vi "crop_with_offset.vi"(0 "Out Rows":i32, 2 "Array":i32[][](array[numeric]), 5 "Out Cols":i32, 9 "Offset X":i32, 11 "Offset Y":i32) -> (4 "subarray":i32[][](array[numeric]))   [LabVIEW 2024]
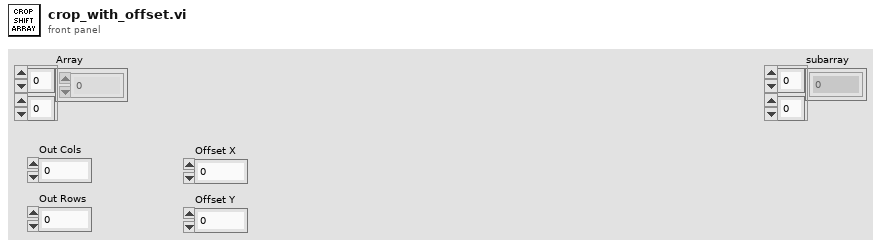
[diagram p1: front panel]
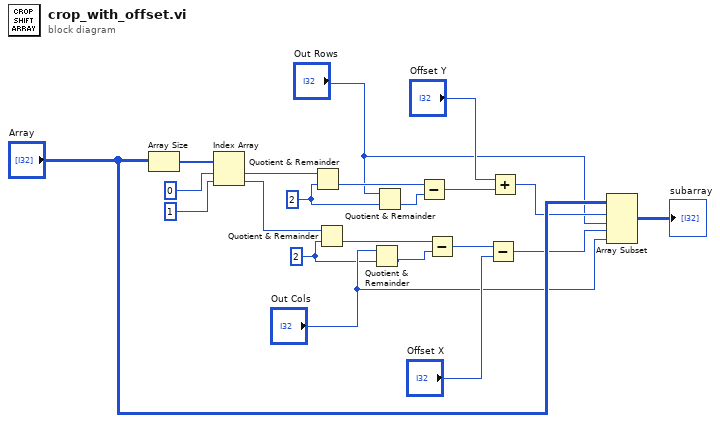
[diagram p0: block diagram]
diagram:
  w2 = 2
  w5 = 2
  n1 = Array Size(array="Array") -> (size(s)=w21:i32[])
  n2 = Index Array(array=w21, index #1=0 ("index"), index #2=1 ("index")) -> (element #1=w18:i32, element #2=w17:i32)
  n3 = Quotient & Remainder(x=w18, y=w5) -> (floor(x/y)=w16:i32)  [unwired: 1 out]
  n4 = Quotient & Remainder(x=w17, y=w2) -> (floor(x/y)=w15:i32)  [unwired: 1 out]
  n5 = Quotient & Remainder(x="Out Cols", y=w2) -> (floor(x/y)=w1:i32)  [unwired: 1 out]
  n6 = Quotient & Remainder(x="Out Rows", y=w5) -> (floor(x/y)=w4:i32)  [unwired: 1 out]
  n7 = Subtract(x=w16, y=w4) -> (x-y=w14:i32)
  n8 = Subtract(x=w15, y=w1) -> (x-y=w13:i32)
  n9 = Subtract(x=w13, y="Offset X") -> (x-y=w10:i32)
  n10 = Add(x="Offset Y", y=w14) -> (x+y=w11:i32)
  n11 = Array Subset(array="Array", index (row)=w11, length (row)="Out Rows", index (col)=w10, length (col)="Out Cols") -> (→"subarray":i32[][])
